vi "weblink create.vi"(5 "[user-specified font]":T1={"Font Name:"="", "Size"=12, "Strikeout?"=FALSE, "Italic?"=FALSE, "Underline?"=FALSE, "Outline?"=FALSE, "Shadow?"=FALSE, "Bold?"=FALSE}, 6 "Force IE? (F)":bool, 7 "desired font(Application)":T2(ring)=enum."Application Font", 8 "error in (no error)":errorcluster, 9 "Link Colors":T4={"Deactivated Color (black)"=0, "Hover Color (blue)"=16860}, 10 "Link Details":T3, 11 "Link Picture Ref (NULL)":refnum<vi>) -> (0 "error out":errorcluster)   [LabVIEW 2011]
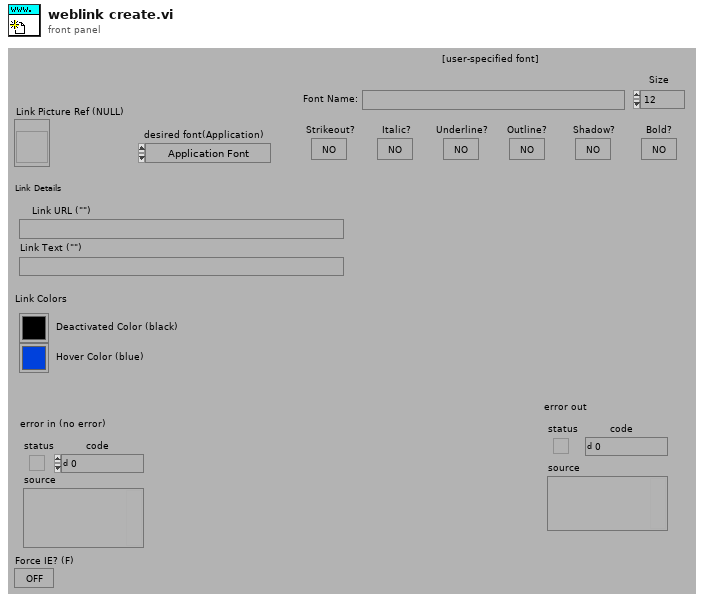
[diagram p1: front panel]
types:
  T1 = cluster{"Font Name:":string, "Size":i16, "Strikeout?":bool, "Italic?":bool, "Underline?":bool, "Outline?":bool, "Shadow?":bool, "Bold?":bool}
  T2 = enum16{"User-specified Font", "Application Font", "System Font", "Dialog Font"}
  T3 = cluster{"Link URL (\"\")":string, "Link Text (\"\")":string}
  T4 = cluster{"Deactivated Color (black)":u32, "Hover Color (blue)":u32}
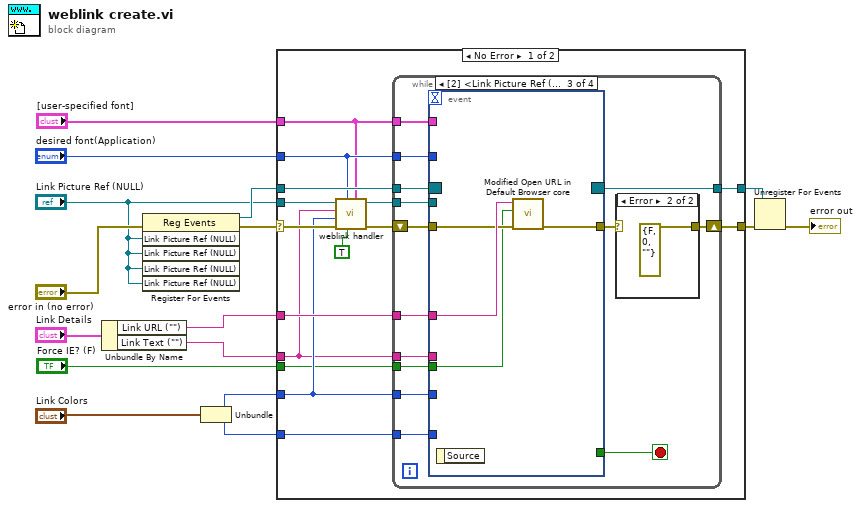
[diagram p0: block diagram]
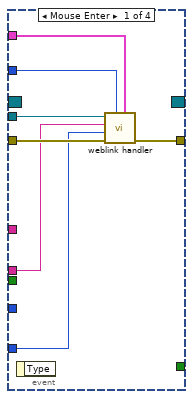
[diagram p3: hidden frame]
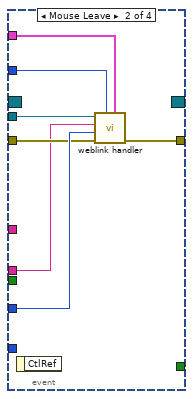
[diagram p4: hidden frame]
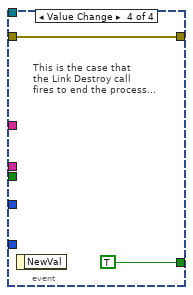
[diagram p5: hidden frame]
diagram:
  n1 = Unbundle By Name("Link Details") -> ("Link URL (\"\")"=w10:string, "Link Text (\"\")"=w9:string)
  n2 = register-events(error in="error in (no error)", "Link Picture Ref (NULL)", "Link Picture Ref (NULL)", "Link Picture Ref (NULL)", "Link Picture Ref (NULL)") -> (reference out=w5:refnum<event-registration>, error out=w15:errorcluster)  [unwired: 1 in]
  n3 = Unbundle("Link Colors") -> ("Deactivated Color (black)"=w13:u32, "Hover Color (blue)"=w12:u32)
  n4 = case shown="No Error" w15 {
    selector: w15 -> [w24 w68]
    tunnel: [w31 w69] -> w16
    tunnel: w12 -> [w30 _]
    tunnel: w5 -> [w29 w69]
    tunnel: w13 -> [w22 _]
    tunnel: w10 -> [w28 _]
    tunnel: "Link Picture Ref (NULL)" -> [w26 _]
    tunnel: w9 -> [w21 _]
    tunnel: [w27 w68] -> w7
    tunnel: "desired font(Application)" -> [w20 _]
    tunnel: "[user-specified font]" -> [w19 _]
    tunnel: "Force IE? (F)" -> [w17 _]
    frame No Error {
      n5 = call "weblink handler.vi"("[user-specified font]"=w19, "Initialize? (f)"=TRUE, "desired font(Application)"=w20, "error in (no error)"=w24, "Link Color (black)"=w22, "Link (\"\")"=w21, "Web\nref"=w26) -> ("error out"=w23:errorcluster, "dup Web\nref"=w25:refnum<vi>)  [unwired: 2 in, 1 out]
      n6 = while {
        tunnel: w25 -> [w44]
        tunnel: [w43] -> w31
        tunnel: w22 -> [w42]
        tunnel: w30 -> [w41]
        tunnel: w28 -> [w40]
        tunnel: w29 -> [w39]
        tunnel: w21 -> [w38]
        shift-right: [w35] -> w27
        shift-left: w23 -> [w37]
        tunnel: w20 -> [w34]
        tunnel: w19 -> [w33]
        tunnel: w17 -> [w32]
        stop <- w45 stop-if-true
        n7 = event shown="[2] <Link Picture Ref (NULL)>: Mouse Down" {
          selector: w39 -> [_ _ _ _]
          dyn-events: [_ _ _ _] -> w43
          timeout: _ -> [_ _ _ _]
          tunnel: w44 -> [w54 w60 _ _]
          tunnel: w41 -> [w50 _ _ _]
          tunnel: w40 -> [_ _ w65 _]
          tunnel: w42 -> [_ w61 _ _]
          tunnel: [_ _ _ TRUE] -> w45
          tunnel: w38 -> [w51 w57 _ _]
          tunnel: w37 -> [w53 w59 w64 w66]
          tunnel: [w52 w58 w63 w66] -> w36
          tunnel: w34 -> [w49 w56 _ _]
          tunnel: w33 -> [w48 w55 _ _]
          tunnel: w32 -> [_ _ w62 _]
          event Mouse Enter {
            n8 = event-data() -> ()  [unwired: 2 out]
            n9 = call "weblink handler.vi"("[user-specified font]"=w48, "desired font(Application)"=w49, "error in (no error)"=w53, "Link Color (black)"=w50, "Link (\"\")"=w51, "Web\nref"=w54) -> ("error out"=w52:errorcluster)  [unwired: 2 in, 3 out]
          }
          event Mouse Leave {
            n10 = event-data() -> ()  [unwired: 2 out]
            n11 = call "weblink handler.vi"("[user-specified font]"=w55, "desired font(Application)"=w56, "error in (no error)"=w59, "Link Color (black)"=w61, "Link (\"\")"=w57, "Web\nref"=w60) -> ("error out"=w58:errorcluster)  [unwired: 3 in, 2 out]
          }
          event Mouse Down {
            n12 = event-data() -> ()  [unwired: 2 out]
            n13 = call "Modified Open URL in Default Browser core.vi"("error in (no error)"=w64, "Force IE? (F)"=w62, "url"=w65) -> ("error out"=w63:errorcluster)  [unwired: 4 out]
          }
          event Value Change {
            # "This is the case that\nthe Link Destroy call\nfires to end the process..."
            n14 = event-data() -> ()  [unwired: 2 out]
          }
        }
        n15 = case shown="Error" w36 {
          selector: w36 -> [w46 _]
          tunnel: [w46 errorcluster {"status"=FALSE, "code"=0, "source"=""} ("error IO")] -> w35
          frame No Error {
          }
          frame Error {
          }
        }
      }
    }
    frame Error {
    }
  }
  n16 = Unregister For Events(event registration refnum=w16, error in=w7) -> (error out=→"error out":errorcluster)
